vi "Read Misc Settings.vi"(4 "Reload":bool, 5 "error in (no error)":errorcluster, 6 "Key":string, 7 "Section":string, 8 "Config Data_Text in":refnum<class "Config Data_Text.lvclass">) -> (0 "error out":errorcluster, 2 "p_value":string, 3 "Config Data_Text out":refnum<class "Config Data_Text.lvclass">)   [LabVIEW 2015, in "Config Data.lvlib" / "Config Data_Text.lvclass"]
uses:
  Config Data_Text.lvclass
  <vilib>/Utility/config.llb/Read Key (String).vi
  <vilib>/Utility/config.llb/Write Key (String).vi
  <vilib>/Utility/config.llb/NI_LVConfig.lvlib
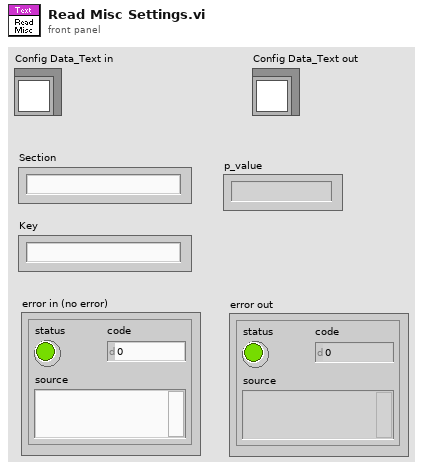
[diagram p1: front panel]
types:
  T1 = typedef "NI_LVConfig.lvlib/Config Data RefNum.ctl" = refnum<k1>
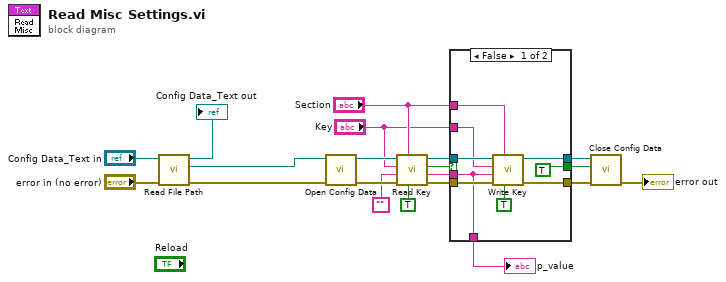
[diagram p0: block diagram]
diagram:
  n1 = call "Read File Path.vi"("Error In"="error in (no error)", "Text In"="Config Data_Text in") -> ("Error Out"=w17:errorcluster, "File Path"=w16:path, "Text Out"=→"Config Data_Text out":refnum<class "Config Data_Text.lvclass">)  [unwired: 3 in]
  n2 = call <vilib>:"Open Config Data.vi"("error in (no error)"=w17, "configuration file path"=w16) -> ("error out"=w15:errorcluster, "refnum"=w14:T1)  [unwired: 7 in, 1 out]
  n3 = call-poly <vilib>:"Read Key.vi"("read raw string? (F)"=TRUE, "section"="Section", "error in (no error)"=w15, "default value"="", "key"="Key", "refnum"=w14) -> ("error out"=w12:errorcluster, "value"=w8:string, "found?"=w9:bool, "refnum out"=w13:T1)  [unwired: 2 in]
  n4 = case shown="False" w9 {
    tunnel: w13 -> [w29 w31]
    tunnel: w12 -> [w28 w30]
    tunnel: w8 -> [w25 w32]
    tunnel: [w25 w32] -> w7
    tunnel: "Section" -> [w22 _]
    tunnel: "Key" -> [w26 _]
    tunnel: [w24 w30] -> w4
    tunnel: [w23 w31] -> w3
    tunnel: [TRUE _] -> w2
    frame False {
      n5 = call-poly <vilib>:"Write Key.vi"("write raw string? (F)"=TRUE ("read raw string? (F)"), "section"=w22, "error in (no error)"=w28, "value"=w25, "key"=w26, "refnum"=w29) -> ("error out"=w24:errorcluster, "refnum out"=w23:T1)  [unwired: 3 in, 1 out]
    }
    frame True {
    }
  }
  "p_value" <- w7
  n6 = call <vilib>:"Close Config Data.vi"("error in (no error)"=w4, "write file if changed (T)"=w2, "refnum"=w3) -> ("error out"=→"error out":errorcluster)  [unwired: 7 in, 1 out]
